vi "Update Status Bar.vi"(8 "Instrument String":string, 9 "Status Bar":refnum<vi>) -> (1 "Status Bar Out":refnum<vi>)   [LabVIEW 2011]
panel:
  out "error out":errorcluster
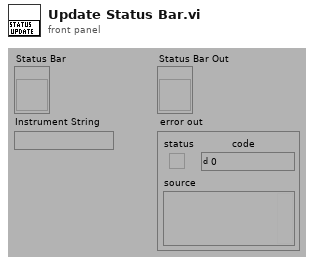
[diagram p1: front panel]
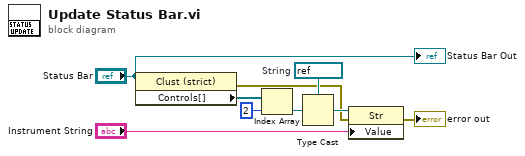
[diagram p0: block diagram]
diagram:
  w7 = refnum<vi> refnum  # String
  n1 = property class="Clust (strict)"(reference="Status Bar") -> (error out=w4:errorcluster, "Controls[]"=w9:refnum<vi>[])  [unwired: 1 in, 1 out]
  n2 = Index Array(array=w9, index=2) -> (element=w6:refnum<vi>)
  n3 = Type Cast(type=w7, x=w6) -> (*(type *) &x=w5:refnum<vi>)
  n4 = property class="Str"(reference=w5, error in=w4, "Value"="Instrument String") -> (error out=→"error out":errorcluster)  [unwired: 1 out]
  "Status Bar Out" <- "Status Bar"
